vi "_Check if Node is Present on BD.vi"(8 "error in (no error)":errorcluster, 9 "Name of Selection":string, 10 "Class Name":T1="Invoke", 11 "path":path) -> (0 "error out":errorcluster, 2 "Found?":bool)   [LabVIEW 2020]
uses:
  _Node Names.ctl
  <vilib>/Utility/traverseref.llb/TRef TravTarget.ctl
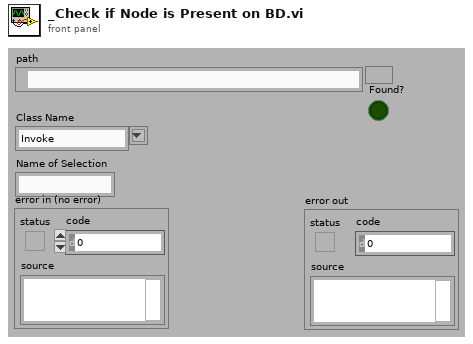
[diagram p1: front panel]
types:
  T1 = typedef "_Node Names.ctl" = string
  T2 = typedef "TRef TravTarget.ctl" = enum16{"FP", "BD", "Other"}
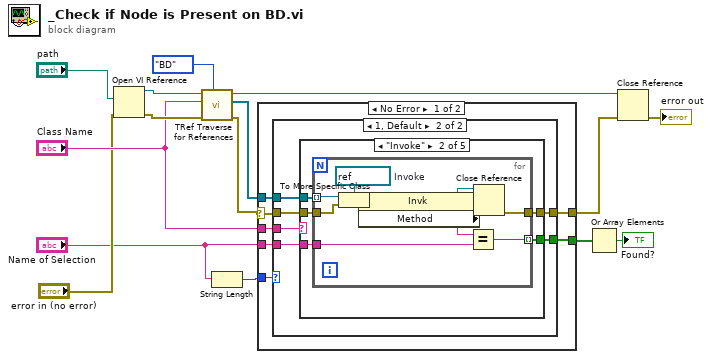
[diagram p0: block diagram]
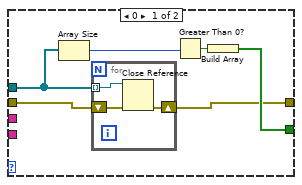
[diagram p2: hidden frame]
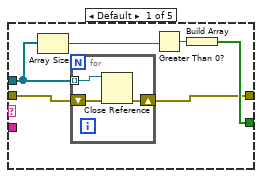
[diagram p3: hidden frame]
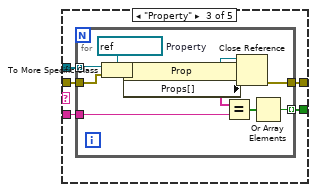
[diagram p4: hidden frame]
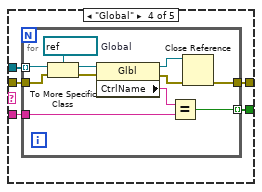
[diagram p5: hidden frame]
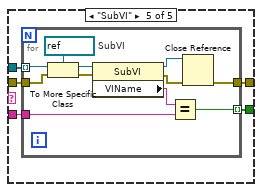
[diagram p6: hidden frame]
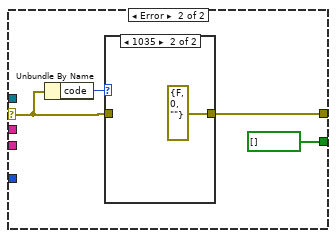
[diagram p7: hidden frame]
diagram:
  n1 = Open VI Reference(vi path="path", error in (no error)="error in (no error)") -> (vi reference=w13:refnum<vi>, error out=w12:errorcluster)  [unwired: 4 in]
  n2 = call <vilib>:"TRef Traverse for References.vi"("Traverse Target"=TRef_TravTarget."BD", "error in (no error)"=w12, "Class Name"="Class Name", "VI Refnum"=w13) -> ("error out"=w1:errorcluster, "References"=w11:refnum<vi>[], "dup VI Refnum"=w7:refnum<vi>)  [unwired: 4 in, 1 out]
  n3 = String Length(string="Name of Selection") -> (length=w3:i32)
  n4 = case shown="No Error" w1 {
    selector: w1 -> [w16 w113]
    tunnel: w11 -> [w22 _]
    tunnel: [w21 bool[] []] -> w10
    tunnel: [w20 w112] -> w8
    tunnel: "Class Name" -> [w19 _]
    tunnel: w3 -> [w18 _]
    tunnel: "Name of Selection" -> [w17 _]
    frame No Error {
      n5 = case shown="1, Default" w18 {
        tunnel: w22 -> [w25 w37]
        tunnel: w17 -> [_ w36]
        tunnel: [w24 w35] -> w21
        tunnel: w16 -> [w26 w34]
        tunnel: [w23 w33] -> w20
        tunnel: w19 -> [_ w32]
        frame 0 {
          n6 = Array Size(array=w25) -> (size(s)=w28:i32)
          n7 = for {
            tunnel: w25 -> [w31] mode=indexing
            shift-right: [w29] -> w23
            shift-left: w26 -> [w30]
            n8 = Close Reference(reference=w31, error in (no error)=w30) -> (error out=w29:errorcluster)
          }
          n9 = Greater Than 0?(x=w28) -> (x > 0?=w27:bool)
          n10 = Build Array(w27) -> (w24:bool[])
        }
        frame 1, Default {
          n11 = case shown="\"Invoke\"" w32 {
            tunnel: w37 -> [w40 w51 w67 w84 w100]
            tunnel: w36 -> [_ w50 w66 w83 w99]
            tunnel: [w41 w49 w65 w82 w98] -> w35
            tunnel: w34 -> [w39 w48 w64 w81 w97]
            tunnel: [w38 w47 w63 w80 w96] -> w33
            frame Default {
              n12 = Array Size(array=w40) -> (size(s)=w43:i32)
              n13 = for {
                tunnel: w40 -> [w46] mode=indexing
                shift-right: [w44] -> w38
                shift-left: w39 -> [w45]
                n14 = Close Reference(reference=w46, error in (no error)=w45) -> (error out=w44:errorcluster)
              }
              n15 = Greater Than 0?(x=w43) -> (x > 0?=w42:bool)
              n16 = Build Array(w42) -> (w41:bool[])
            }
            frame "Invoke" {
              n17 = for {
                tunnel: w51 -> [w61] mode=indexing
                tunnel: w50 -> [w59]
                tunnel: [w58] -> w49 mode=indexing
                tunnel: w48 -> [w57]
                tunnel: [w53] -> w47
                w62 = refnum<vi> refnum  # Invoke
                n18 = To More Specific Class(target class=w62, reference=w61, error in=w57) -> (specific class reference=w60:refnum<vi>, error out=w56:errorcluster)
                n19 = property class="Invk"(reference=w60, error in=w56) -> (reference out=w54:refnum<vi>, error out=w55:errorcluster, "Method"=w52:string)
                n20 = Equal?(x=w52, y=w59) -> (x = y?=w58:bool)
                n21 = Close Reference(reference=w54, error in (no error)=w55) -> (error out=w53:errorcluster)
              }
            }
            frame "Property" {
              n22 = for {
                tunnel: w67 -> [w78] mode=indexing
                tunnel: w66 -> [w76]
                tunnel: [w68] -> w65 mode=indexing
                tunnel: w64 -> [w74]
                tunnel: [w70] -> w63
                w79 = refnum<vi> refnum  # Property
                n23 = To More Specific Class(target class=w79, reference=w78, error in=w74) -> (specific class reference=w77:refnum<vi>, error out=w73:errorcluster)
                n24 = property class="Prop"(reference=w77, error in=w73) -> (reference out=w71:refnum<vi>, error out=w72:errorcluster, "Props[]"=w69:string[])
                n25 = Equal?(x=w69, y=w76) -> (x = y?=w75:bool[])
                n26 = Close Reference(reference=w71, error in (no error)=w72) -> (error out=w70:errorcluster)
                n27 = Or Array Elements(Boolean array=w75) -> (logical OR=w68:bool)
              }
            }
            frame "Global" {
              n28 = for {
                tunnel: w84 -> [w94] mode=indexing
                tunnel: w83 -> [w92]
                tunnel: [w85] -> w82 mode=indexing
                tunnel: w81 -> [w91]
                tunnel: [w87] -> w80
                w95 = refnum<vi> refnum  # Global
                n29 = To More Specific Class(target class=w95, reference=w94, error in=w91) -> (specific class reference=w93:refnum<vi>, error out=w90:errorcluster)
                n30 = property class="Glbl"(reference=w93, error in=w90) -> (reference out=w88:refnum<vi>, error out=w89:errorcluster, "CtrlName"=w86:string)
                n31 = Equal?(x=w86, y=w92) -> (x = y?=w85:bool)
                n32 = Close Reference(reference=w88, error in (no error)=w89) -> (error out=w87:errorcluster)
              }
            }
            frame "SubVI" {
              n33 = for {
                tunnel: w100 -> [w110] mode=indexing
                tunnel: w99 -> [w108]
                tunnel: [w101] -> w98 mode=indexing
                tunnel: w97 -> [w107]
                tunnel: [w103] -> w96
                w111 = refnum<vi> refnum  # SubVI
                n34 = To More Specific Class(target class=w111, reference=w110, error in=w107) -> (specific class reference=w109:refnum<vi>, error out=w106:errorcluster)
                n35 = property class="SubVI"(reference=w109, error in=w106) -> (reference out=w104:refnum<vi>, error out=w105:errorcluster, "VIName"=w102:string)
                n36 = Equal?(x=w102, y=w108) -> (x = y?=w101:bool)
                n37 = Close Reference(reference=w104, error in (no error)=w105) -> (error out=w103:errorcluster)
              }
            }
          }
        }
      }
    }
    frame Error {
      n38 = Unbundle By Name(w113) -> ("code"=w114:i32)
      n39 = case shown="1035" w114 {
        tunnel: w113 -> [w116 _]
        tunnel: [w116 errorcluster {"status"=FALSE, "code"=0, "source"=""} ("error IO")] -> w112
        frame 0, Default {
        }
        frame 1035 {
        }
      }
    }
  }
  n40 = Or Array Elements(Boolean array=w10) -> (logical OR=→"Found?":bool)
  n41 = Close Reference(reference=w7, error in (no error)=w8) -> (error out=→"error out":errorcluster)
